vi "Join.vi"(0 "Axis":string, 3 "Controller #":u8=1, 4 "Joystick buttons":T1={"MinDir"=1, "MaxDir"=2, "MedSpeed"=5, "HighSpeed"=6} {"HighSpeed" min=1 max=25 step=1; "MedSpeed" min=1 max=25 step=1; "MaxDir" min=1 max=25 step=1; "MinDir" min=1 max=25 step=1}, 5 "error in":errorcluster, 6 "Primary Zaber":T2={"Serial port handle"="", "Axis"="", "Controller #"=0, "Min position"=0.0, "Max position"=0.0, "Min velocity"=0.0, "Max velocity"=0.0, "Firmware"="", "Device ID"=0, "Variable event"=refnum, "Variable ref"=refnum, "Resolution, usteps/step"=0, "Serial port semaphore"=refnum, "Joystick buttons"={"MinDir"=1, "MaxDir"=2, "MedSpeed"=5, "HighSpeed"=6}} {"Joystick buttons"."HighSpeed" min=1 max=25 step=1; "Joystick buttons"."MedSpeed" min=1 max=25 step=1; "Joystick buttons"."MaxDir" min=1 max=25 step=1; "Joystick buttons"."MinDir" min=1 max=25 step=1}) -> (14 "Zaber":T2={"Serial port handle"="", "Axis"="", "Controller #"=0, "Min position"=0.0, "Max position"=0.0, "Min velocity"=0.0, "Max velocity"=0.0, "Firmware"="", "Device ID"=0, "Variable event"=refnum, "Variable ref"=refnum, "Resolution, usteps/step"=0, "Serial port semaphore"=refnum, "Joystick buttons"={"MinDir"=1, "MaxDir"=2, "MedSpeed"=5, "HighSpeed"=6}} {"Joystick buttons"."HighSpeed" min=1 max=25 step=1; "Joystick buttons"."MedSpeed" min=1 max=25 step=1; "Joystick buttons"."MaxDir" min=1 max=25 step=1; "Joystick buttons"."MinDir" min=1 max=25 step=1}, 19 "error out":errorcluster)   [LabVIEW 2018]
uses:
  Zaber.ctl
  GenericDataEvent/GenericEvent.ctl
  ZaberVariables.ctl
  Stage joystick buttons.ctl
  GenericDataEvent/GenericData.ctl
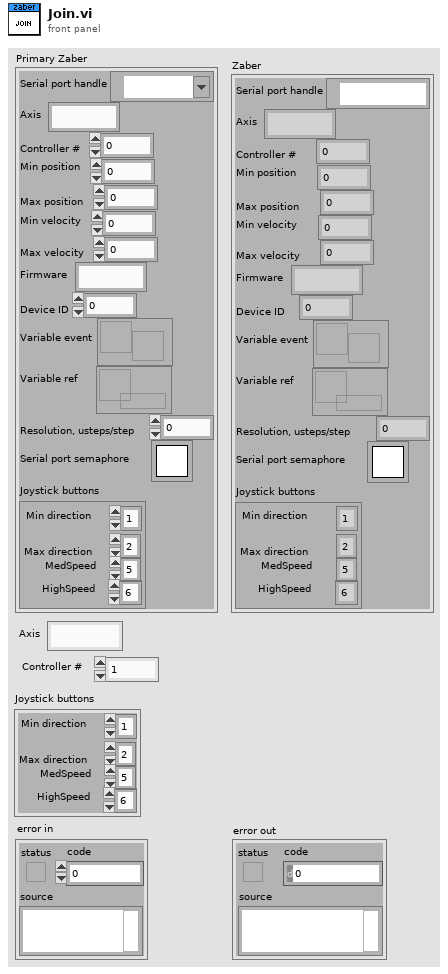
[diagram p1: front panel]
types:
  T1 = typedef "Stage joystick buttons.ctl" = cluster{"MinDir":i32, "MaxDir":i32, "MedSpeed":i32, "HighSpeed":i32}
  T2 = typedef "Zaber.ctl" = cluster{"Serial port handle":refnum<visa-resource-name>, "Axis":string, "Controller #":u8, "Min position":dbl, "Max position":dbl, "Min velocity":dbl, "Max velocity":dbl, "Firmware":string, "Device ID":i32, "Variable event":T3, "Variable ref":refnum<data-value>, "Resolution, usteps/step":i32, "Serial port semaphore":T4, "Joystick buttons":cluster{"MinDir":i32, "MaxDir":i32, "MedSpeed":i32, "HighSpeed":i32}}
  T3 = typedef "GenericEvent.ctl" = refnum<user-event>
  T4 = typedef "Semaphore RefNum" = refnum<k1>
  T5 = typedef "ZaberVariables.ctl" = cluster{"Position":i32, "Speed":i32, "Min soft position":dbl, "Max soft position":dbl, "Accelaration":i32}
  T6 = typedef "GenericData.ctl" = cluster{"Name":string, "Data":variant}
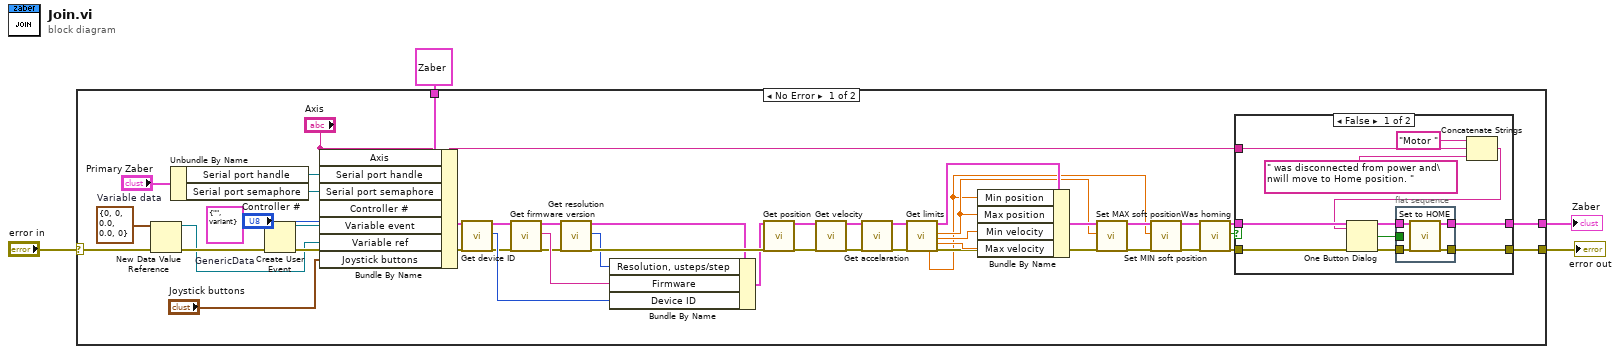
[diagram p0: block diagram]
diagram:
  n1 = case shown="No Error" "error in" {
    selector: "error in" -> [w29 w68]
    tunnel: [w27 w68] -> w1
    tunnel: [w26 w67] -> w2
    tunnel: T2 {"Serial port handle"="", "Axis"="", "Controller #"=0, "Min position"=0.0, "Max position"=0.0, "Min velocity"=0.0, "Max velocity"=0.0, "Firmware"="", "Device ID"=0, "Variable event"=refnum, "Variable ref"=refnum, "Resolution, usteps/step"=0, "Serial port semaphore"=refnum, "Joystick buttons"={"MinDir"=1, "MaxDir"=2, "MedSpeed"=5, "HighSpeed"=6}} ("Zaber") -> [w51 w67]
    frame No Error {
      w7 = T5 {"Position"=0, "Speed"=0, "Min soft position"=0.0, "Max soft position"=0.0, "Accelaration"=0}  # Variable data
      w40 = T6 {"Name"="", "Data"=variant}  # GenericData
      n2 = New Data Value Reference(data value=w7, error in=w29) -> (data value reference=w28:refnum<data-value>, error out=w30:errorcluster)
      n3 = Unbundle By Name("Primary Zaber") -> ("Serial port handle"=w42:refnum<visa-resource-name>, "Serial port semaphore"=w15:T4)
      n4 = Create User Event(user event datatype=w40, error in=w30) -> (user event=w37:refnum<user-event>, error out=w38:errorcluster)
      n5 = Bundle By Name(cluster=w51, "Axis"="Axis", "Serial port handle"=w42, "Serial port semaphore"=w15, "Controller #"="Controller #", "Variable event"=w37, "Variable ref"=w28, "Joystick buttons"="Joystick buttons") -> (w41:T2)
      n6 = call "Get device ID.vi"("Zaber"=w41, "error in"=w38) -> ("Zaber out"=w22:T2, "Device ID"=w24:i32, "error out"=w23:errorcluster)  [unwired: 15 in]
      n7 = call "Get firmware version.vi"("Zaber"=w22, "error in"=w23) -> ("Zaber out"=w19:T2, "Firmware version"=w25:string, "error out"=w20:errorcluster)  [unwired: 15 in]
      n8 = call "Get resolution.vi"("Zaber in"=w19, "error in"=w20) -> ("Zaber out"=w18:T2, "Resolution, usteps/step"=w16:u16, "error out"=w21:errorcluster)  [unwired: 15 in]
      n9 = Bundle By Name(cluster=w18, "Resolution, usteps/step"=w16, "Firmware"=w25, "Device ID"=w24) -> (w17:T2)
      n10 = call "Get position.vi"("Zaber"=w17, "error in"=w21) -> ("Zaber out"=w35:T2, "error out"=w36:errorcluster)  [unwired: 13 in, 3 out]
      n11 = call "Get velocity.vi"("Zaber"=w35, "error in"=w36) -> ("Zaber out"=w31:T2, "error out"=w34:errorcluster)  [unwired: 14 in, 2 out]
      n12 = call "Get accelaration.vi"("Zaber"=w31, "error in"=w34) -> ("Zaber out"=w32:T2, "error out"=w33:errorcluster)  [unwired: 14 in, 2 out]
      n13 = call "Get limits.vi"("Zaber"=w32, "error in"=w33) -> ("MIN position, mm"=w6:dbl, "Zaber out"=w50:T2, "MAX position, mm"=w8:dbl, "MIN velociry, mm/s"=w49:dbl, "MAX velocity, mm/s"=w48:dbl, "error out"=w12:errorcluster)  [unwired: 11 in, 1 out]
      n14 = Bundle By Name(cluster=w50, "Min position"=w6, "Max position"=w8, "Min velocity"=w49, "Max velocity"=w48) -> (w10:T2)
      n15 = call "Set MAX soft position.vi"("Zaber"=w10, "Max soft position"=w8, "error in"=w12) -> ("Zaber out"=w13:T2, "error out"=w14:errorcluster)  [unwired: 14 in, 1 out]
      n16 = call "Set MIN soft position.vi"("Zaber"=w13, "Min soft position"=w6, "error in"=w14) -> ("Zaber out"=w9:T2, "error out"=w11:errorcluster)  [unwired: 14 in, 1 out]
      n17 = call "Was homing.vi"("Zaber"=w9, "error in"=w11) -> ("Zaber out"=w47:T2, "Was homing?"=w45:bool, "error out"=w46:errorcluster)  [unwired: 15 in]
      n18 = case shown="False" w45 {
        tunnel: w46 -> [w59 w65]
        tunnel: [w58 w65] -> w27
        tunnel: w47 -> [w57 w66]
        tunnel: [w56 w66] -> w26
        tunnel: "Axis" -> [w54 _]
        frame False {
          n19 = flat-sequence {
            tunnel: w60 -> [_]
            tunnel: w59 -> [w64]
            tunnel: [w63] -> w58
            tunnel: w57 -> [w62]
            tunnel: [w61] -> w56
            frame #0 {
              n20 = call "Set to HOME.vi"("Zaber"=w62, "error in"=w64) -> ("Zaber out"=w61:T2, "error out"=w63:errorcluster)  [unwired: 16 in]
            }
          }
          n21 = Concatenate Strings("Motor " ("string"), w54, " was disconnected from power and\nwill move to Home position. " ("message")) -> (w52:string)
          n22 = One Button Dialog(message=w52) -> (true=w60:bool)  [unwired: 1 in]
        }
        frame True {
        }
      }
    }
    frame Error {
    }
  }
  "error out" <- w1
  "Zaber" <- w2
